vi "Lesson 3 Launcher.vi"() -> ()   [LabVIEW 2020]
panel:
  out "error out":errorcluster
  out "error out Process":errorcluster
  out "error out AQN":errorcluster
  in  "error in":errorcluster
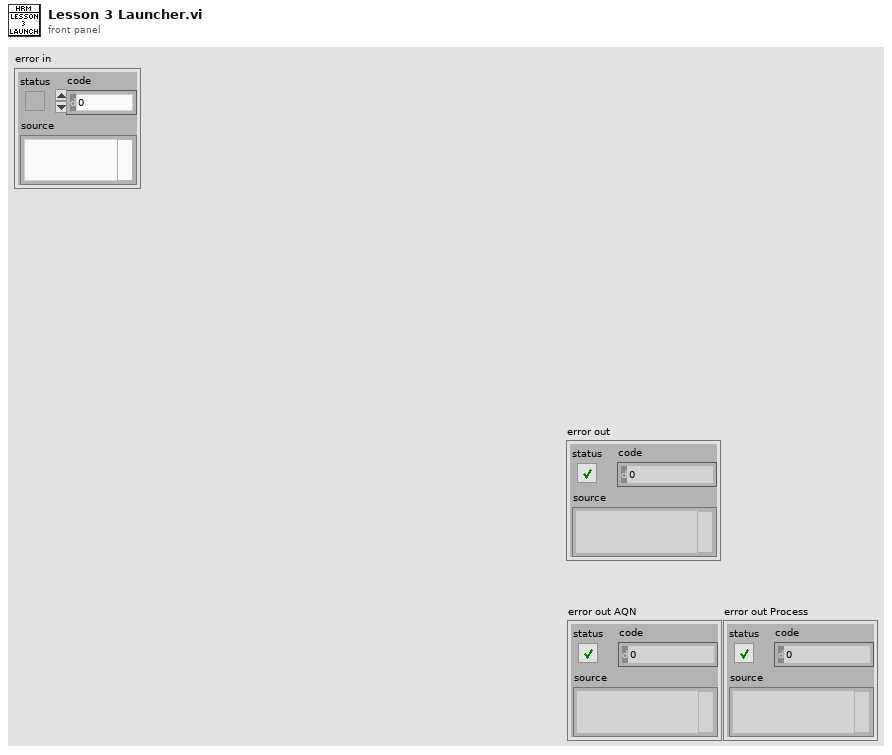
[diagram p1: front panel]
types:
  T1 = typedef "HRM-init-cluster.ctl" = cluster{"User Events":T2}
  T2 = typedef "HRM-init-user_events.ctl" = cluster{"Additional Signal to remove [s]":refnum<user-event>, "samples [s]":refnum<user-event>, "Heart Rate":refnum<user-event>, "Raw collected data":refnum<user-event>, "Filtered data":refnum<user-event>, "Raw Data":refnum<user-event>, "stop":refnum<user-event>}
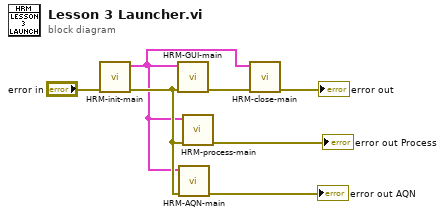
[diagram p0: block diagram]
diagram:
  n1 = call "HRM-init-main.vi"("error in (no error)"="error in") -> ("error out"=w7:errorcluster, "init cluster"=w2:T1)  [unwired: 9 in]
  n2 = call "HRM-GUI-main.vi"("error in (no error)"=w7, "init cluster"=w2) -> ("error out"=w1:errorcluster)  [unwired: 9 in]
  n3 = call "HRM-AQN-main.vi"("error in (no error)"=w7, "init cluster"=w2) -> ("error out"=→"error out AQN":errorcluster)  [unwired: 9 in]
  n4 = call "HRM-process-main.vi"("error in (no error)"=w7, "init cluster"=w2) -> ("error out"=→"error out Process":errorcluster)  [unwired: 9 in]
  n5 = call "HRM-close-main.vi"("error in (no error)"=w1, "init cluster"=w2) -> ("error out"=→"error out":errorcluster)  [unwired: 9 in]
